vi "test_VISAFactory_InitializeMeasurementLinkSessionWithInitAndClose_RemoteSessionCreatedAndClosed.vi"(8 "error in":errorcluster) -> (0 "error out":errorcluster, 2 "result":string, 3 "pass":bool)   [LabVIEW 2020, in "MeasurementServerTests.lvlib"]
uses:
  MeasurementServerTests.lvlib
  Runtime/Sessions/Instrument/ISession Factory/Initialize and Close Session Behavior.ctl
  Runtime/Sessions/Instrument/ISession Factory/ISession Factory.lvclass
  Runtime/Sessions/VISA/Session Factory/Session Factory.lvclass
  <vilib>/Instr/_visa.llb/VISA Open Access Mode.ctl
  <vilib>/NI-VISA/VISA gRPC Open Close Behavior.ctl
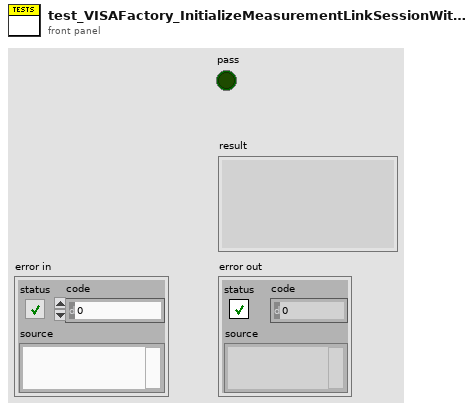
[diagram p1: front panel]
types:
  T1 = typedef "VISA Open Access Mode.ctl" = u32
  T2 = typedef "NI Session Management Instrument.lvlib/ISession Factory.lvclass/Remote Connection Options.ctl" = cluster{"session name":string, "address":string, "port":u32}
  T3 = typedef "VISA gRPC Open Close Behavior.ctl" = enum16{"Auto", "Initialize and Close", "Attach and Detach", "Initialize and Detach", "Attach and Close"}
  T4 = typedef "NI Session Management Instrument.lvlib/ISession Factory.lvclass/Initialize and Close Session Behavior.ctl" = enum16{"Initialize and Close", "Attach and Detach", "Initialize and Detach", "Attach and Close"}
  T5 = typedef "NI Session Management Instrument.lvlib/ISession Factory.lvclass/Session Initialization Parameters.ctl" = cluster{"resource name":string, "session name":string}
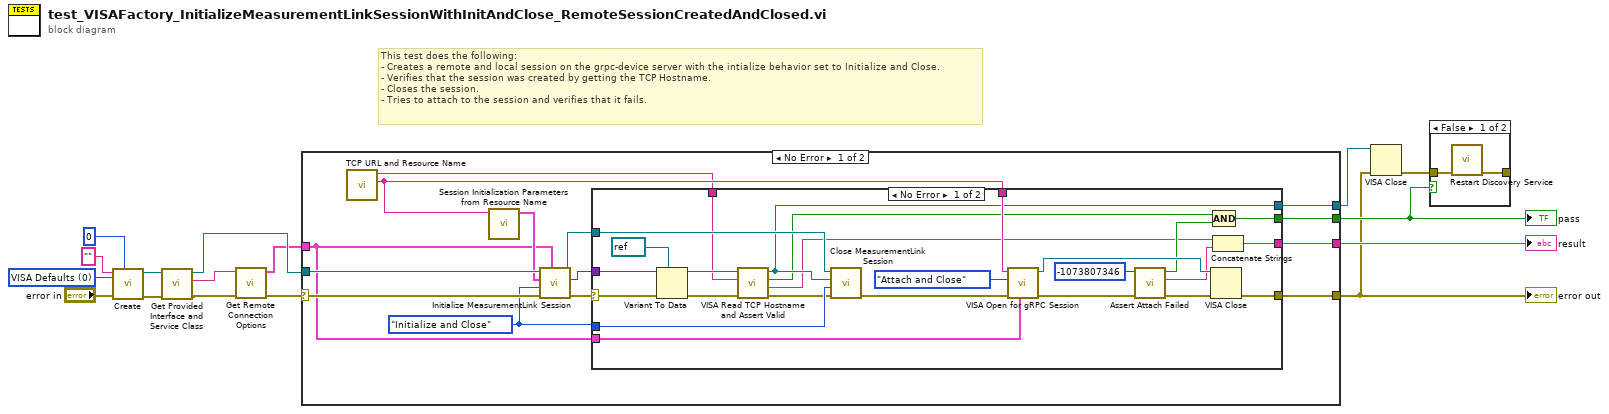
[diagram p0: block diagram]
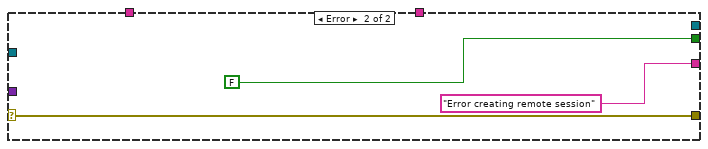
[diagram p2: hidden frame]
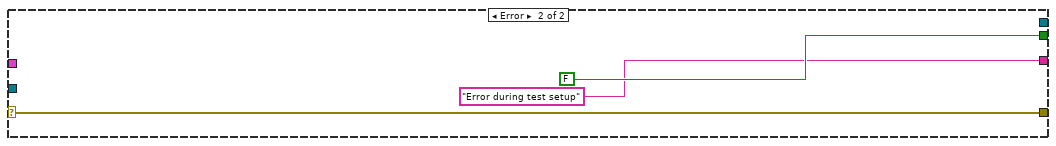
[diagram p3: hidden frame]
diagram:
  w2 = T1 0 items=["VISA Defaults"=0, "Exclusive Lock"=1, "Load Configured Settings"=4] ("access mode")
  # "This test does the following:\n- Creates a remote and local session on the grpc-device server with the intialize behavior set to Initialize and Close.\n- Verifies that the session was created by getting the TCP Hostname.\n- Closes the session.\n- Tries to attach to the session and verifies that it fails."
  n1 = call "Create.vi"("visa open timeout"=u32 0, "error in"="error in", "access mode"=w2, "instrument type id"="") -> ("error out"=w7:errorcluster, "session factory out"=w6:refnum<class "Session Factory.lvclass">)  [unwired: 6 in]
  n2 = call-dynamic "Get Provided Interface and Service Class.vi"("error in"=w7, "session factory in"=w6) -> ("error out"=w8:errorcluster, "provided interface"=w5:string, "session factory out"=w9:refnum<class "Session Factory.lvclass">)  [unwired: 6 in, 1 out]
  n3 = call "Get Remote Connection Options.vi"("error in"=w8, "provided interface"=w5) -> ("error out"=w15:errorcluster, "remote connection options"=w1:T2)  [unwired: 8 in]
  n4 = case shown="No Error" w15 {
    selector: w15 -> [w25 w59]
    tunnel: [w29 w59] -> w11
    tunnel: [w30 FALSE] -> w12
    tunnel: [w28 "Error during test setup" ("f")] -> w16
    tunnel: w1 -> [w19 _]
    tunnel: w9 -> [w24 _]
    tunnel: [w23 _] -> w14
    frame No Error {
      w20 = Initialize_and_Close_Session_Behavior."Initialize and Close" ("initialize and close session behavior")
      n5 = call "TCP URL and Resource Name.vi"() -> ("visa resource name"=w18:string, "url"=w17:string)  [unwired: 10 in]
      n6 = call "Session Initialization Parameters from Resource Name.vi"("resource name"=w18) -> ("session initialization parameters"=w22:T5)  [unwired: 10 in]
      n7 = call-dynamic "Initialize MeasurementLink Session.vi"("remote connection options"=w19, "error in"=w25, "initialize and close session behavior"=w20, "session initialization parameters"=w22, "session factory in"=w24) -> ("error out"=w26:errorcluster, "session out"=w27:variant, "session factory out"=w21:refnum<class "Session Factory.lvclass">)  [unwired: 4 in]
      n8 = case shown="No Error" w26 {
        selector: w26 -> [w54 w57]
        tunnel: [w52 FALSE] -> w30
        tunnel: [w44 w57] -> w29
        tunnel: [w51 "Error creating remote session"] -> w28
        tunnel: w27 -> [w55 _]
        tunnel: [w34 _] -> w23
        tunnel: w21 -> [w50 _]
        tunnel: w20 -> [w49 _]
        tunnel: w18 -> [w47 _]
        tunnel: w19 -> [w43 _]
        tunnel: w17 -> [w35 _]
        frame No Error {
          n9 = Variant To Data(error in=w54, type=refnum<visa-resource-name> refnum ("VISA resource name out"), Variant=w55) -> (data=w36:refnum<visa-resource-name>, error out=w37:errorcluster)
          n10 = call "VISA Read TCP Hostname and Assert Valid.vi"("error in"=w37, "expected hostname"=w35, "visa refnum in"=w36) -> ("error out"=w31:errorcluster, "result"=w32:string, "pass?"=w33:bool, "visa refnum out"=w34:refnum<visa-resource-name>)  [unwired: 5 in]
          n11 = call-dynamic "Close MeasurementLink Session.vi"("error in"=w31, "initialize and close session behavior"=w49, "session in"=w34, "session factory in"=w50) -> ("error out"=w48:errorcluster)  [unwired: 7 in]
          n12 = call <vilib>:"VISA Open for gRPC Session.vi"("gRPC Options"=w43, "error in (no error)"=w48, "open/close behavior"=VISA_gRPC_Open_Close_Behavior."Attach and Close" ("Open/Close Behavior"), "VISA resource name"=w47) -> ("error out"=w42:errorcluster, "VISA resource name out"=w45:refnum<visa-resource-name>)  [unwired: 6 in]
          n13 = call "Assert Attach Failed.vi"("error in"=w42, "attach error code"=-1073807346) -> ("error out"=w41:errorcluster, "result"=w40:string, "pass?"=w39:bool)  [unwired: 7 in]
          n14 = VISA Close(VISA resource name=w45, error in (no error)=w41) -> (error out=w44:errorcluster)
          n15 = Compound Arithmetic op=AND(w33, w39) -> (w52:bool)
          n16 = Concatenate Strings(w32, w40) -> (w51:string)
        }
        frame Error {
        }
      }
    }
    frame Error {
    }
  }
  "error out" <- w11
  "pass" <- w12
  "result" <- w16
  n17 = VISA Close(VISA resource name=w14, error in (no error)=w11) -> (error out=w13:errorcluster)
  n18 = case shown="False" w12 {
    tunnel: w13 -> [w63 _]
    tunnel: [w62 _] -> _
    frame False {
      n19 = call "Restart Discovery Service.vi"("error in"=w63) -> ("error out"=w62:errorcluster)  [unwired: 10 in]
    }
    frame True {
    }
  }
